vi "Cut Waveform with Cursors.vi"(10 "CrsrList":T1, 11 "Waveform in":waveform(dbl)) -> (2 "Td":dbl, 3 "Waveform out":waveform(dbl))   [LabVIEW 2014, in "Aquisicao de Dados.lvlib"]
uses:
  Aquisicao de Dados.lvlib
  <vilib>/Utility/miscctls.llb/LVCursorListTypeDef.ctl
  <vilib>/Waveform/WDTOps.llb/WDT Get Waveform Subset DBL.vi
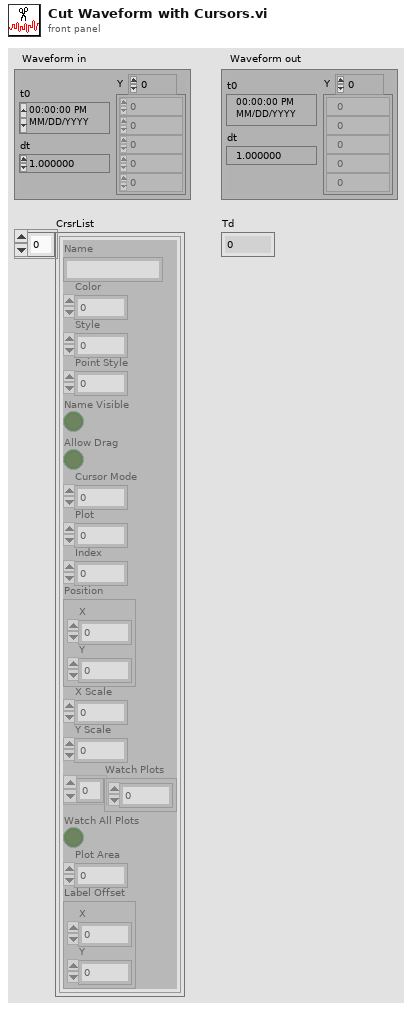
[diagram p1: front panel]
types:
  T1 = typedef "LVCursorListTypeDef.ctl" = cluster{"Name":string, "Color":u32, "Style":u8, "Point Style":u8, "Name Visible":bool, "Allow Drag":bool, "Cursor Mode":u32, "Plot":i32, "Index":i32, "Position":cluster{"X":dbl, "Y":dbl}, "X Scale":u32, "Y Scale":u32, "Watch Plots":i32[], "Watch All Plots":bool, "Plot Area":i32, "Label Offset":cluster{"X":dbl, "Y":dbl}}[]
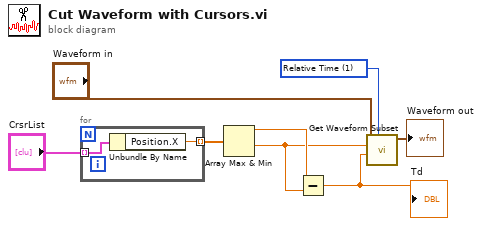
[diagram p0: block diagram]
diagram:
  w5 = u16 1 items=["Samples", "Relative Time"] ("start/duration format")
  n1 = for {
    tunnel: "CrsrList" -> [w10] mode=indexing
    tunnel: [w9] -> w8 mode=indexing
    n2 = Unbundle By Name(w10) -> ("Position.X"=w9:dbl)
  }
  n3 = Array Max & Min(array=w8) -> (max value=w6:dbl, min value=w4:dbl)  [unwired: 2 out]
  n4 = Subtract(x=w6, y=w4) -> (x-y=w7:dbl)
  "Td" <- w7
  n5 = call-poly <vilib>:"Get Waveform Subset.vi"("start/duration format"=w5, "duration"=w7, "start samples/time"=w4, "waveform in"="Waveform in") -> ("waveform out"=→"Waveform out":waveform(dbl))  [unwired: 2 in, 3 out]
